vi "caraRG.vi"() -> ()   [LabVIEW 2020]
panel:
  out "new picture":picture
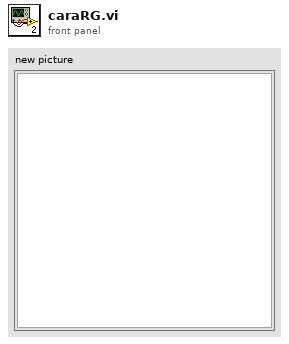
[diagram p1: front panel]
types:
  T1 = typedef "imagedata.ctl" = cluster{"image type":i32, "image depth":i32, "image":u8[], "mask":u8[], "colors":u32[], "Rectangle":cluster{"left":i16, "top":i16, "right":i16, "bottom":i16}}
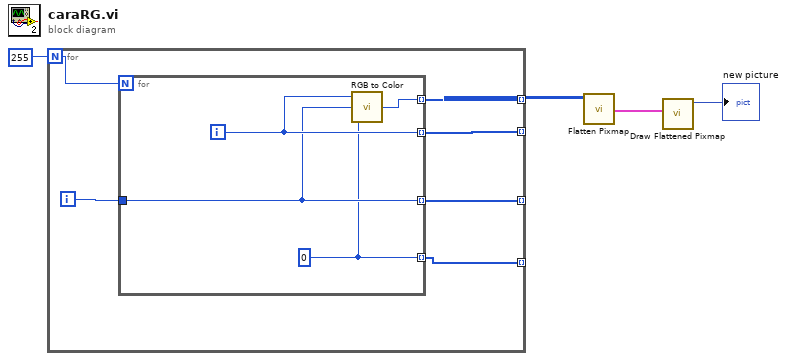
[diagram p0: block diagram]
diagram:
  n1 = for {
    N: 255 -> [w6]
    tunnel: [w10] -> _ mode=indexing
    tunnel: [w8] -> _ mode=indexing
    tunnel: [w7] -> _ mode=indexing
    tunnel: [w5] -> w3 mode=indexing
    i -> [w9]
    n2 = for {
      N: w6 -> [_]
      tunnel: [w14] -> w10 mode=indexing
      tunnel: w9 -> [w13]
      tunnel: [w13] -> w8 mode=indexing
      tunnel: [w12] -> w7 mode=indexing
      tunnel: [w11] -> w5 mode=indexing
      i -> [w14]
      w12 = 0
      n3 = call <vilib>:"RGB to Color.vi"("B"=w12, "G"=w13, "R"=w14) -> ("Color"=w11:u32)
    }
  }
  n4 = call <vilib>:"Flatten Pixmap.vi"("24-bit pixmap"=w3) -> ("image data"=w2:T1)  [unwired: 10 in]
  n5 = call <vilib>:"Draw Flattened Pixmap.vi"("image data"=w2) -> ("new picture"=→"new picture":picture)  [unwired: 8 in]
